vi "NOx parse MAX win.vi"() -> (0 "NOx output array":dbl[](array[numeric]))   [LabVIEW 2011]
panel:
  out "NOxSensorData 2":T1={"NOx (ppm)"=0, "O2 (%)"=0.0, "Sensor Supply Status"=3, "Sensor Temperature Status"=12, "NOx Signal Status"=48, "O2 Signal Status"=192, "Heater Mode Status"=96, "Heater Circuit Status"=31, "NOx Circuit Status"=31, "O2 Circuit Status"=31, "NOx Sensor Module Present"=FALSE} {"Heater Mode Status" items=["AUTO MODE"=0, "HEATUP SLOPE 3 OR 4"=32, "HEATUP SLOPE 1 OR 2"=64, "HEATER OFF / PREHEAT"=96]; "O2 Circuit Status" items=["OPEN WIRE"=3, "SHORT CIRCUIT"=5, "NO ERROR"=31]; "NOx Circuit Status" items=["OPEN WIRE"=3, "SHORT CIRCUIT"=5, "NO ERROR"=31]; "Heater Circuit Status" items=["OPEN WIRE"=3, "SHORT CIRCUIT"=5, "NO ERROR"=31]; "Sensor Temperature Status" items=["NOT AT TEMPERATURE"=0, "AT TEMPERATURE"=4, "ERROR"=8, "NOT AVAILABLE"=12]; "O2 Signal Status" items=["NOT VALID"=0, "VALID"=64, "ERROR"=128, "NOT AVAILABLE"=192]; "NOx Signal Status" items=["NOT VALID"=0, "VALID"=16, "ERROR"=32, "NOT AVAILABLE"=48]; "Sensor Supply Status" items=["NOT IN RANGE", "SUPPLY IN RANGE", "ERROR", "NOT AVAILABLE"]}
  out "NOxSensorData 1":T1={"NOx (ppm)"=0, "O2 (%)"=0.0, "Sensor Supply Status"=3, "Sensor Temperature Status"=12, "NOx Signal Status"=48, "O2 Signal Status"=192, "Heater Mode Status"=96, "Heater Circuit Status"=31, "NOx Circuit Status"=31, "O2 Circuit Status"=31, "NOx Sensor Module Present"=FALSE} {"Heater Mode Status" items=["AUTO MODE"=0, "HEATUP SLOPE 3 OR 4"=32, "HEATUP SLOPE 1 OR 2"=64, "HEATER OFF / PREHEAT"=96]; "O2 Circuit Status" items=["OPEN WIRE"=3, "SHORT CIRCUIT"=5, "NO ERROR"=31]; "NOx Circuit Status" items=["OPEN WIRE"=3, "SHORT CIRCUIT"=5, "NO ERROR"=31]; "Heater Circuit Status" items=["OPEN WIRE"=3, "SHORT CIRCUIT"=5, "NO ERROR"=31]; "Sensor Temperature Status" items=["NOT AT TEMPERATURE"=0, "AT TEMPERATURE"=4, "ERROR"=8, "NOT AVAILABLE"=12]; "O2 Signal Status" items=["NOT VALID"=0, "VALID"=64, "ERROR"=128, "NOT AVAILABLE"=192]; "NOx Signal Status" items=["NOT VALID"=0, "VALID"=16, "ERROR"=32, "NOT AVAILABLE"=48]; "Sensor Supply Status" items=["NOT IN RANGE", "SUPPLY IN RANGE", "ERROR", "NOT AVAILABLE"]}
  in  "NOxSensorDataFromFPGA 1":T2={"NOx (bits)"=0, "O2 (bits)"=0, "Sensor Supply Status"=3, "Sensor Temperature Status"=12, "NOx Signal Status"=48, "O2 Signal Status"=192, "Heater Mode Status"=96, "Heater Circuit Status"=31, "NOx Circuit Status"=31, "O2 Circuit Status"=31, "NOx Sensor Module Present"=FALSE} {"Heater Mode Status" items=["AUTO MODE"=0, "HEATUP SLOPE 3 OR 4"=32, "HEATUP SLOPE 1 OR 2"=64, "HEATER OFF / PREHEAT"=96]; "O2 Circuit Status" items=["OPEN WIRE"=3, "SHORT CIRCUIT"=5, "NO ERROR"=31]; "NOx Circuit Status" items=["OPEN WIRE"=3, "SHORT CIRCUIT"=5, "NO ERROR"=31]; "Heater Circuit Status" items=["OPEN WIRE"=3, "SHORT CIRCUIT"=5, "NO ERROR"=31]; "Sensor Temperature Status" items=["NOT AT TEMPERATURE"=0, "AT TEMPERATURE"=4, "ERROR"=8, "NOT AVAILABLE"=12]; "O2 Signal Status" items=["NOT VALID"=0, "VALID"=64, "ERROR"=128, "NOT AVAILABLE"=192]; "NOx Signal Status" items=["NOT VALID"=0, "VALID"=16, "ERROR"=32, "NOT AVAILABLE"=48]; "Sensor Supply Status" items=["NOT IN RANGE", "SUPPLY IN RANGE", "ERROR", "NOT AVAILABLE"]}
  in  "NOxSensorDataFromFPGA 2":T2={"NOx (bits)"=0, "O2 (bits)"=0, "Sensor Supply Status"=3, "Sensor Temperature Status"=12, "NOx Signal Status"=48, "O2 Signal Status"=192, "Heater Mode Status"=96, "Heater Circuit Status"=31, "NOx Circuit Status"=31, "O2 Circuit Status"=31, "NOx Sensor Module Present"=FALSE} {"Heater Mode Status" items=["AUTO MODE"=0, "HEATUP SLOPE 3 OR 4"=32, "HEATUP SLOPE 1 OR 2"=64, "HEATER OFF / PREHEAT"=96]; "O2 Circuit Status" items=["OPEN WIRE"=3, "SHORT CIRCUIT"=5, "NO ERROR"=31]; "NOx Circuit Status" items=["OPEN WIRE"=3, "SHORT CIRCUIT"=5, "NO ERROR"=31]; "Heater Circuit Status" items=["OPEN WIRE"=3, "SHORT CIRCUIT"=5, "NO ERROR"=31]; "Sensor Temperature Status" items=["NOT AT TEMPERATURE"=0, "AT TEMPERATURE"=4, "ERROR"=8, "NOT AVAILABLE"=12]; "O2 Signal Status" items=["NOT VALID"=0, "VALID"=64, "ERROR"=128, "NOT AVAILABLE"=192]; "NOx Signal Status" items=["NOT VALID"=0, "VALID"=16, "ERROR"=32, "NOT AVAILABLE"=48]; "Sensor Supply Status" items=["NOT IN RANGE", "SUPPLY IN RANGE", "ERROR", "NOT AVAILABLE"]}
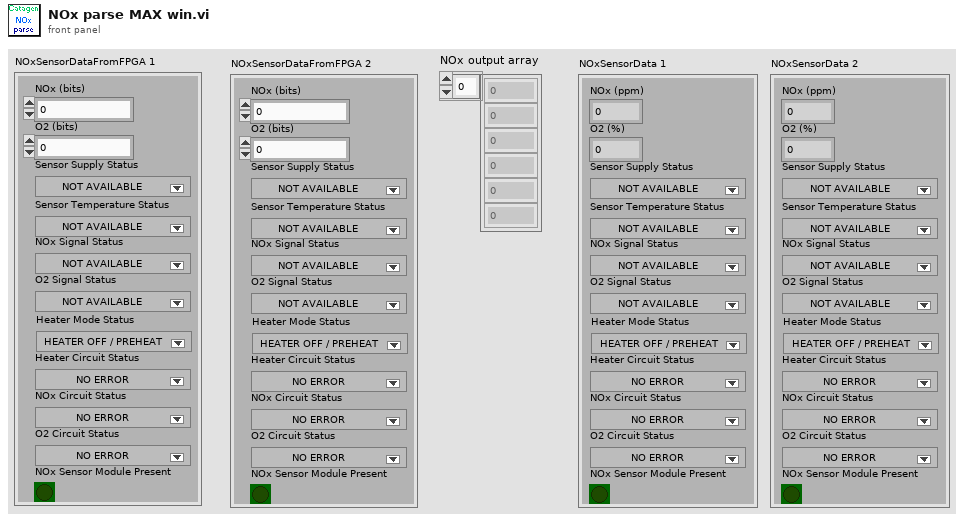
[diagram p1: front panel]
types:
  T1 = cluster{"NOx (ppm)":i16, "O2 (%)":sgl, "Sensor Supply Status":u8, "Sensor Temperature Status":u8, "NOx Signal Status":u8, "O2 Signal Status":u8, "Heater Mode Status":u8, "Heater Circuit Status":u8, "NOx Circuit Status":u8, "O2 Circuit Status":u8, "NOx Sensor Module Present":bool}
  T2 = cluster{"NOx (bits)":i16, "O2 (bits)":u16, "Sensor Supply Status":u8, "Sensor Temperature Status":u8, "NOx Signal Status":u8, "O2 Signal Status":u8, "Heater Mode Status":u8, "Heater Circuit Status":u8, "NOx Circuit Status":u8, "O2 Circuit Status":u8, "NOx Sensor Module Present":bool}
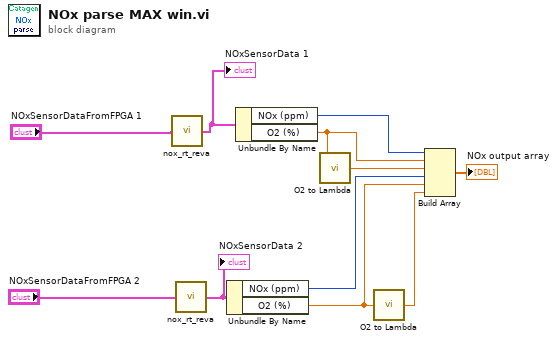
[diagram p0: block diagram]
diagram:
  n1 = call <vilib>:"nox_rt_reva.vi"("NOxSensorDataFromFPGA"="NOxSensorDataFromFPGA 1") -> ("NOxSensorData"=w3:T1)
  "NOxSensorData 1" <- w3
  n2 = call <vilib>:"nox_rt_reva.vi"("NOxSensorDataFromFPGA"="NOxSensorDataFromFPGA 2") -> ("NOxSensorData"=w1:T1)
  "NOxSensorData 2" <- w1
  n3 = Unbundle By Name(w1) -> ("NOx (ppm)"=w8:i16, "O2 (%)"=w7:sgl)
  n4 = Unbundle By Name(w3) -> ("NOx (ppm)"=w11:i16, "O2 (%)"=w10:sgl)
  n5 = call "O2 to Lambda.vi"("O2 %"=w10) -> ("Lambda"=w9:dbl)
  n6 = call "O2 to Lambda.vi"("O2 %"=w7) -> ("Lambda"=w6:dbl)
  n7 = Build Array(w11, w10, w9, w8, w7, w6) -> (→"NOx output array":dbl[])
